vi "Get_measurement_samplingdata.vi"(0 "SPU":refnum<k24>, 1 "Meas_monitor_struct":refnum<k24>[](array[refnum]), 2 "MPM":refnum<k24>[](array[refnum]), 3 "TSL":refnum<k24>, 4 "Data_struct":refnum<k24>[](array[refnum]), 5 "错误输入（无错误）":errorcluster, 6 "STSProcess.PDLSTS":refnum<k24>, 7 "SweepCount":i32, 11 "SOP":i32) -> (19 "error out":errorcluster)   [LabVIEW 2017]
doc: "Get logging measurement data & add in"
uses:
  D:/test/PDLSTS/LV_PDL LvVer17.0/LV_PDL_x64/DLL/STSProcess.dll
  DLL/STSProcess.dll
  D:/test/PDLSTS/LV_PDL LvVer17.0/LV_PDL_x64/DLL/InstrumentDLL.dll
  DLL/InstrumentDLL.dll
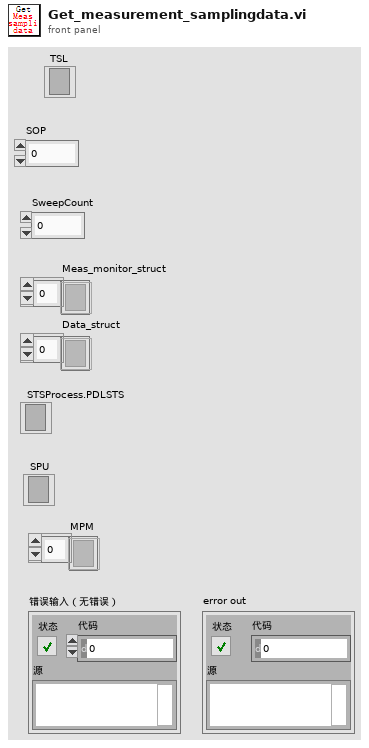
[diagram p1: front panel]
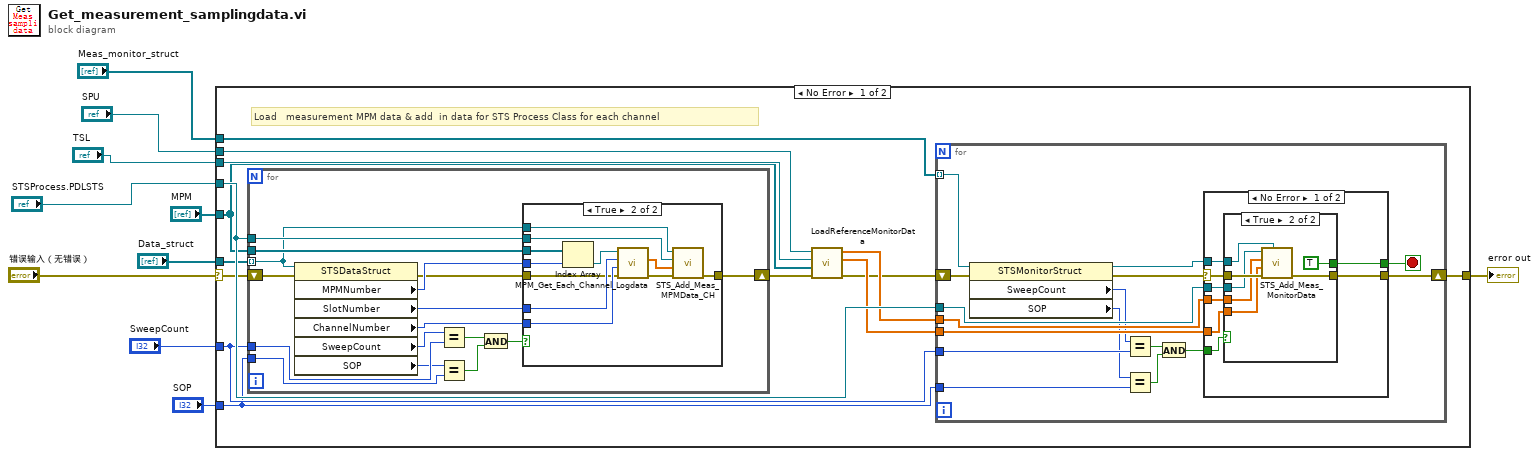
[diagram p0: block diagram]
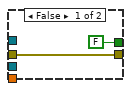
[diagram p2: hidden frame]
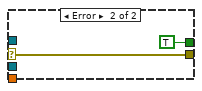
[diagram p3: hidden frame]
diagram:
  n1 = case shown="No Error" "错误输入（无错误）" {
    selector: "错误输入（无错误）" -> [w20 w88]
    tunnel: "STSProcess.PDLSTS" -> [w24 _]
    tunnel: "Meas_monitor_struct" -> [w23 _]
    tunnel: "SPU" -> [w14 _]
    tunnel: "MPM" -> [w11 _]
    tunnel: "Data_struct" -> [w22 _]
    tunnel: [w21 w88] -> w7
    tunnel: "SweepCount" -> [w19 _]
    tunnel: "SOP" -> [w18 _]
    tunnel: "TSL" -> [w12 _]
    frame No Error {
      # "Load　measurement MPM data & add  in data for STS Process Class for each channel"
      n2 = for {
        tunnel: w22 -> [w67] mode=indexing
        tunnel: w11 -> [w73]
        tunnel: w24 -> [w68]
        tunnel: w19 -> [w65]
        shift-right: [w69] -> w13
        shift-left: w20 -> [w70]
        tunnel: w18 -> [w63]
        n3 = property on="属性节点" class="STSDataStruct"(reference=w67, error in=w70) -> (error out=w71:errorcluster, "MPMNumber"=w72:i32, "SlotNumber"=w75:i32, "ChannelNumber"=w74:i32, "SweepCount"=w66:i32, "SOP"=w64:i32)  [unwired: 1 out]
        n4 = Equal?(x=w66, y=w65) -> (x = y?=w62:bool)
        n5 = Equal?(x=w64, y=w63) -> (x = y?=w61:bool)
        n6 = And(x=w62, y=w61) -> (x .and. y?=w60:bool)
        n7 = case shown="True" w60 {
          tunnel: w75 -> [_ w87]
          tunnel: w74 -> [_ w86]
          tunnel: w73 -> [_ w85]
          tunnel: w72 -> [_ w84]
          tunnel: w71 -> [w76 w83]
          tunnel: [w76 w81] -> w69
          tunnel: w68 -> [_ w78]
          tunnel: w67 -> [_ w77]
          frame False {
          }
          frame True {
            n8 = Index Array(array=w85, index=w84) -> (element=w82:refnum<k24>)
            n9 = call "MPM_Get_Each_Channel_Logdata.vi"("error in (no error)"=w83, "channelNumber"=w86, "moduleNumber"=w87, ".NET Reference in"=w82) -> ("error out"=w80:errorcluster, "data out"=w79:sgl[])  [unwired: 5 in, 1 out]
            n10 = call "STS_Add_Meas_MPMData_CH.vi"("错误输入（无错误）"=w80, "data"=w79, "STSProcess.PDLSTS"=w78, ".NET引用句柄输入"=w77) -> ("错误输出"=w81:errorcluster)  [unwired: 6 in, 1 out]
          }
        }
      }
      n11 = call "LoadReferenceMonitorData.vi"("错误输入（无错误）"=w13, "MPM"=w11, "TSL"=w12, "SPU"=w14) -> ("错误输出"=w15:errorcluster, "monitor"=w16:sgl[], "trigger"=w17:sgl[])  [unwired: 5 in]
      n12 = for {
        tunnel: w23 -> [w36] mode=indexing
        tunnel: w24 -> [w40]
        tunnel: w17 -> [w39]
        tunnel: w16 -> [w38]
        shift-right: [w37] -> w21
        shift-left: w15 -> [w32]
        tunnel: w19 -> [w34]
        tunnel: w18 -> [w29]
        stop <- w25 stop-if-true
        n13 = property on="属性节点" class="STSMonitorStruct"(reference=w36, error in=w32) -> (reference out=w33:refnum<k24>, error out=w31:errorcluster, "SweepCount"=w35:i32, "SOP"=w30:i32)
        n14 = Equal?(x=w35, y=w34) -> (x = y?=w28:bool)
        n15 = Equal?(x=w30, y=w29) -> (x = y?=w27:bool)
        n16 = And(x=w28, y=w27) -> (x .and. y?=w26:bool)
        n17 = case shown="No Error" w31 {
          selector: w31 -> [w47 w59]
          tunnel: w40 -> [w46 _]
          tunnel: w33 -> [w43 _]
          tunnel: w39 -> [w45 _]
          tunnel: w38 -> [w44 _]
          tunnel: [w48 w59] -> w37
          tunnel: w26 -> [w42 _]
          tunnel: [w41 TRUE] -> w25
          frame No Error {
            n18 = case shown="True" w42 {
              tunnel: [w50 w57] -> w48
              tunnel: w47 -> [w50 w56]
              tunnel: w46 -> [_ w55]
              tunnel: w45 -> [_ w54]
              tunnel: w44 -> [_ w53]
              tunnel: w43 -> [_ w52]
              tunnel: [FALSE TRUE] -> w41
              frame False {
              }
              frame True {
                n19 = call "STS_Add_Meas_MonitorData.vi"("setting"=w52, "错误输入（无错误）"=w56, "monitorData"=w53, "triggerIndex"=w54, "STSProcess.PDLSTS"=w55) -> ("错误输出"=w57:errorcluster)  [unwired: 5 in, 1 out]
              }
            }
          }
          frame Error {
          }
        }
      }
    }
    frame Error {
    }
  }
  "error out" <- w7
